vi "WL_XNET_Globals.vi"() -> ()   [LabVIEW 2021]
panel:
  out "DBC_Settings_Write":T1={"ByteOrder"=[enum."Motorola", enum."Motorola"], "Type"=[], "Factor"=[1.0, 1.0], "Offset"=[0.0, 0.0], "Startbit"=[27, 43], "Length"=[16, 16], "Mux"=[FALSE, FALSE], "Name"=["", ""]} {"Offset" format="%.3f"; "Factor" format="%.3f"}
  out "DBC_Settings_Complete":T1={"ByteOrder"=[enum."Motorola", enum."Motorola"], "Type"=[], "Factor"=[1.0, 1.0], "Offset"=[0.0, 0.0], "Startbit"=[27, 43], "Length"=[16, 16], "Mux"=[FALSE, FALSE], "Name"=["", ""]} {"Offset" format="%.3f"; "Factor" format="%.3f"}
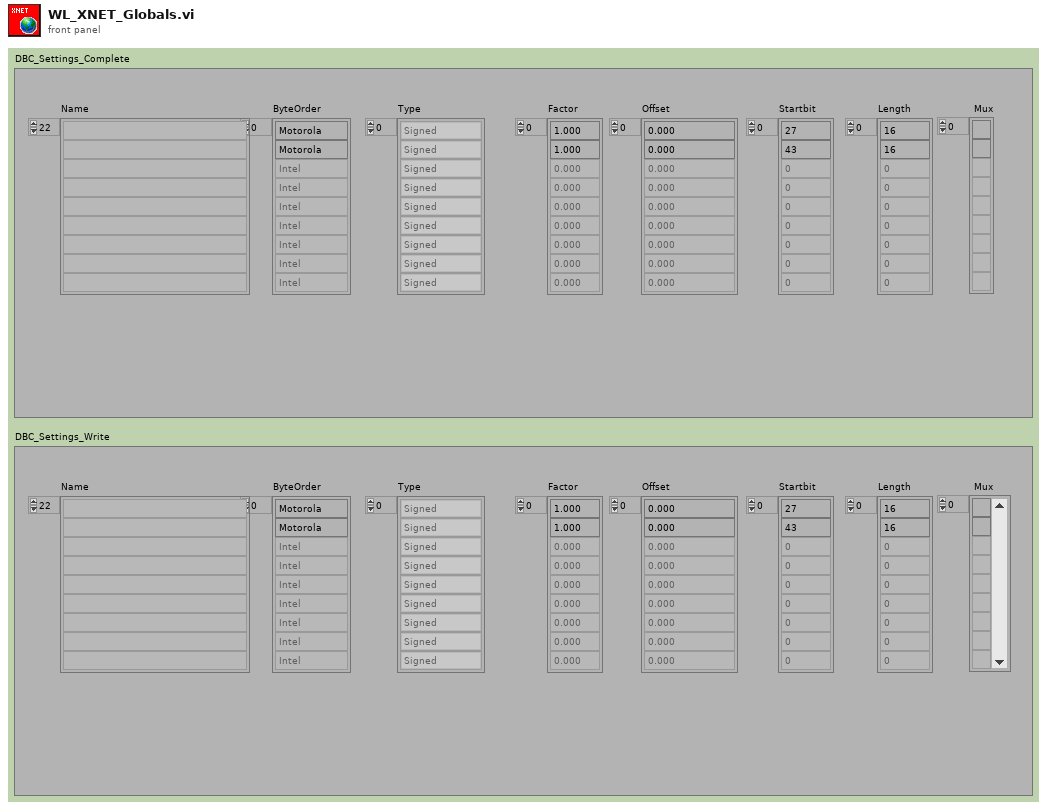
[diagram p1: front panel]
types:
  T1 = cluster{"ByteOrder":enum16{"Intel", "Motorola"}[], "Type":enum16{"Signed", "Unsigned", "IEEE Float", "Byte Array"}[], "Factor":dbl[], "Offset":dbl[], "Startbit":u32[], "Length":u32[], "Mux":bool[], "Name":string[]}
diagram:
